vi "ukol4.vi"() -> ()   [LabVIEW 2023]
uses:
  <vilib>/Analysis/2dsp.llb/Real FFT.vi
  <vilib>/Utility/file.llb/Read Delimited Spreadsheet (DBL).vi
  <vilib>/Analysis/NI_AALPro.lvlib
panel:
  out "x-y":dbl
  out "Waveform Graph 3":waveform(dbl)(graph)
  out "Waveform Graph 2":waveform(dbl)(graph)
  out "Waveform Graph":waveform(dbl)(graph)
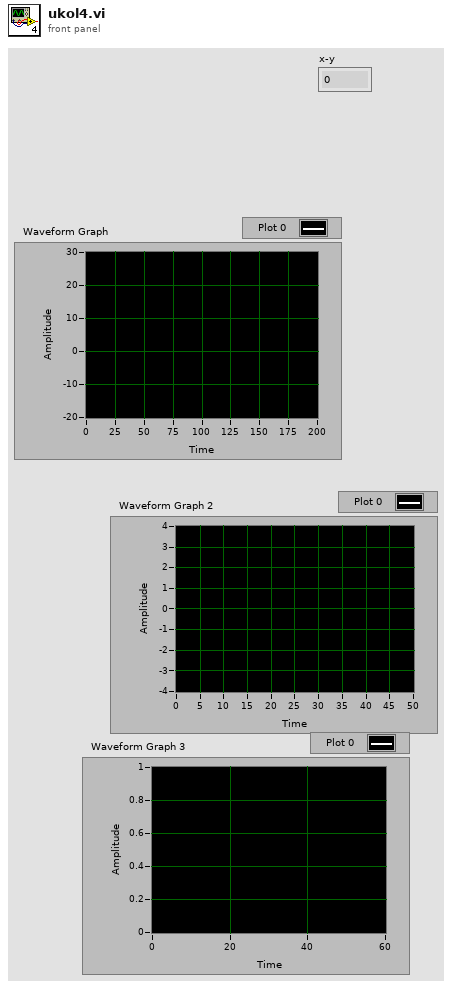
[diagram p1: front panel]
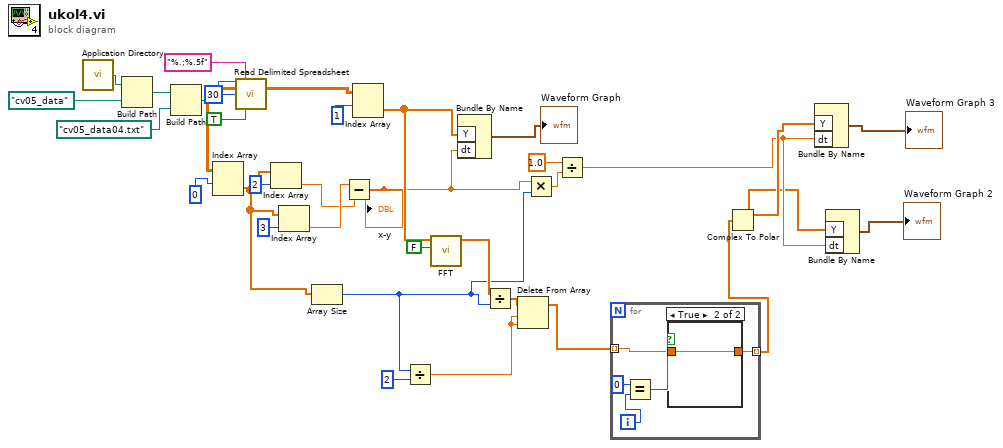
[diagram p0: block diagram]
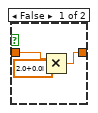
[diagram p2: hidden frame]
diagram:
  n1 = call <vilib>:"Application Directory.vi"() -> ("Application Directory"=w34:path)
  n2 = Build Path(base path=w34, name or relative path=path "cv05_data") -> (appended path=w32:path)
  n3 = Build Path(base path=w32, name or relative path=path "cv05_data04.txt") -> (appended path=w30:path)
  n4 = call-poly <vilib>:"Read Delimited Spreadsheet.vi"("file path (dialog if empty)"=w30, "format (%.3f)"="%.;%.5f", "start of read offset (chars.:0)"=30, "transpose? (F)"=TRUE) -> ("all rows"=w20:dbl[][])  [unwired: 6 in, 5 out]
  n5 = Index Array(array=w20, index (row)=0) -> (element=w19:dbl[])  [unwired: 1 in]
  n6 = Index Array(array=w19, index=2) -> (element=w7:dbl)
  n7 = Index Array(array=w19, index=3) -> (element=w8:dbl)
  n8 = Array Size(array=w19) -> (size(s)=w11:i32)
  n9 = Subtract(x=w8, y=w7) -> (x-y=w12:dbl)
  "x-y" <- w12
  n10 = Index Array(array=w20, index (row)=1) -> (element=w24:dbl[])  [unwired: 1 in]
  n11 = Divide(x=w11, y=2) -> (x/y=w14:dbl)
  n12 = call-poly <vilib>:"FFT.vi"("shift?"=FALSE, "X"=w24) -> ("FFT {X}"=w22:cdb[])  [unwired: 8 in, 1 out]
  n13 = Bundle By Name("Y"=w24, "dt"=w12) -> (→"Waveform Graph":waveform(dbl))  [unwired: 1 in]
  n14 = Divide(x=w22, y=w11) -> (x/y=w16:cdb[])
  n15 = Delete From Array(array=w16, length=w14, index=w14) -> (array with subset deleted=w2:cdb[])  [unwired: 1 out]
  n16 = Multiply(x=w12, y=w11) -> (x*y=w5:dbl)
  n17 = Divide(x=1.0, y=w5) -> (x/y=w4:dbl)
  n18 = for {
    tunnel: w2 -> [w35] mode=indexing
    tunnel: [w36] -> w1 mode=indexing
    i -> [w39]
    n19 = Equal?(x=0, y=w39) -> (x = y?=w37:bool)
    n20 = case shown="True" w37 {
      tunnel: [w40 w43] -> w36
      tunnel: w35 -> [w42 w43]
      frame False {
        n21 = Multiply(x=w42, y=cdb 2.0+0.0i) -> (x*y=w40:cdb)
      }
      frame True {
      }
    }
  }
  n22 = Complex To Polar(r * e^(i*theta)=w1) -> (r=w10:dbl[], theta=w3:dbl[])
  n23 = Bundle By Name("Y"=w10, "dt"=w4) -> (→"Waveform Graph 3":waveform(dbl))  [unwired: 1 in]
  n24 = Bundle By Name("Y"=w3, "dt"=w4) -> (→"Waveform Graph 2":waveform(dbl))  [unwired: 1 in]
